vi "optionsAcq_cycleCountingWavemeter.vi"(0 "reference":refnum<class "OSA200.lvclass">, 2 "cycleCounting":bool, 4 "readWrite":enum16{"read", "write"}(ring), 5 "error in (no error)":errorcluster, 7 "ignore range violation (false)":bool) -> (14 "duplicate reference":refnum<class "OSA200.lvclass">, 15 "status":string, 16 "cycleCounting out":bool, 19 "error out":errorcluster)   [LabVIEW 2010, in "OSA200.lvclass"]
doc: "Enable/disable cyclecounting of interferogram.\n\nSee also"
uses:
  OSA200.lvclass
  OSA.lvclass
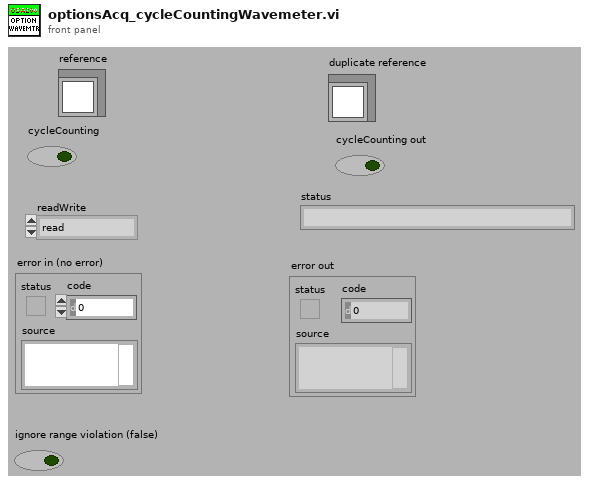
[diagram p1: front panel]
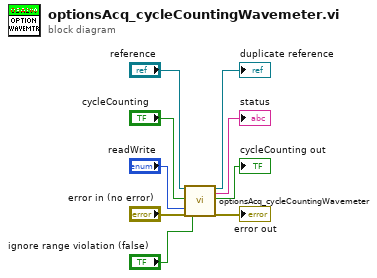
[diagram p0: block diagram]
diagram:
  n1 = call-parent "optionsAcq_cycleCountingWavemeter.vi"("reference"="reference", "cycleCounting"="cycleCounting", "readWrite"="readWrite", "error in (no error)"="error in (no error)", "ignore range violation (false)"="ignore range violation (false)") -> ("duplicate reference"=→"duplicate reference":refnum<class "OSA200.lvclass">, "status"=→"status":string, "cycleCounting out"=→"cycleCounting out":bool, "error out"=→"error out":errorcluster)  [unwired: 11 in]
